vi "Global_Line-Fake.vi"() -> ()   [LabVIEW 2017, in "Hopper System.lvlib"]
uses:
  Hopper System.lvlib
panel:
  out "Line Sensor-Fake_Testor":bool
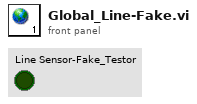
[diagram p1: front panel]
diagram:
